vi "test_generic.vi"() -> ()   [LabVIEW 2010, in "GenericObjective.lvclass"]
uses:
  GenericObjective.lvclass
  common/classes/XMLElement/XMLElement/XMLElement.lvclass
  common/classes/GenericComponent/GenericComponent/GenericComponent.lvclass
panel:
  in  "configure button":bool
  in  "stop button":bool
  in  "create OME XML button":bool
  out "OME XML":string
  in  "createButton":bool
  # "Test program for Objective components"
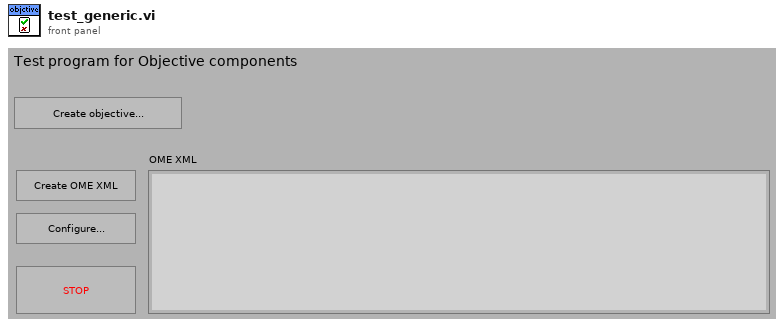
[diagram p1: front panel]
types:
  T1 = typedef "XComponentSpecification.xctl/data.ctl" = cluster{"class path":string, "configuration":string, "label":string, "settings name":string}
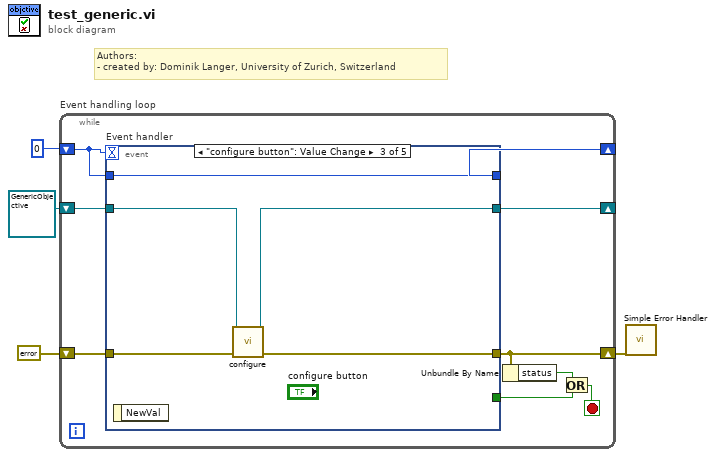
[diagram p0: block diagram]
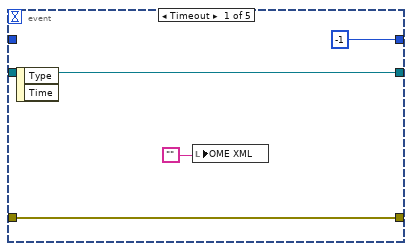
[diagram p2: hidden frame]
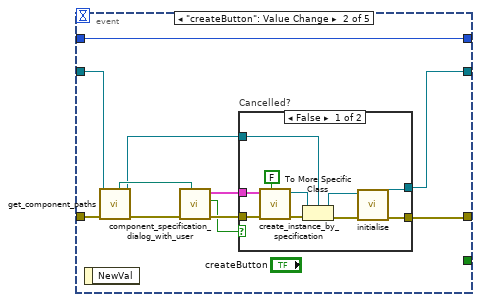
[diagram p3: hidden frame]
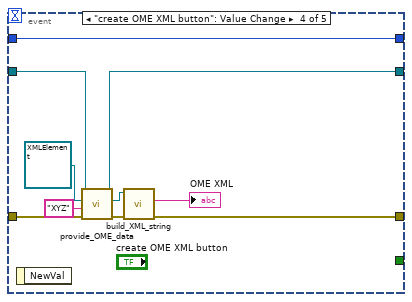
[diagram p5: hidden frame]
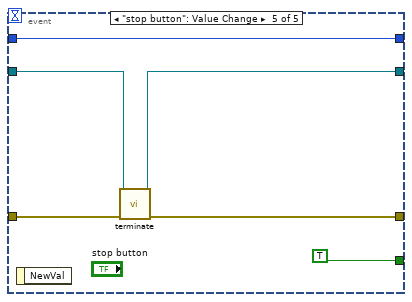
[diagram p6: hidden frame]
diagram:
  # "Authors: \n- created by: Dominik Langer, University of Zurich, Switzerland"
  n1 = while "Event handling loop" {
    shift-right: [w8] -> w1
    shift-left: errorcluster {"status"=FALSE, "code"=0, "source"=""} ("error out") -> [w13]
    shift-right: [w11] -> _
    shift-left: 0 -> [w12]
    shift-right: [w10] -> _
    shift-left: refnum<class "GenericObjective.lvclass"> refnum ("GenericObjective.lvclass") -> [w9]
    stop <- w6 stop-if-true
    n2 = event "Event handler" shown="[2] \"configure button\": Value Change" {
      selector: _ -> [_ _ _ _ _]
      dyn-events: _ -> [_ _ _ _ _]
      timeout: w12 -> [_ _ _ _ _]
      tunnel: w13 -> [w14 w21 w44 w54 w59]
      tunnel: [w14 w27 w43 w47 w58] -> w8
      tunnel: [-1 w28 w45 w55 w61] -> w11
      tunnel: w12 -> [_ w28 w45 w55 w61]
      tunnel: [w15 w26 w41 w52 w56] -> w10
      tunnel: w9 -> [w15 w23 w42 w53 w57]
      tunnel: [_ _ _ _ TRUE] -> w5
      event Timeout {
        n3 = event-data() -> ()  [unwired: 1 in, 2 out]
        n4 = local write "OME XML"("") -> ()
      }
      event "createButton": Value Change {
        n5 = event-data() -> ()  [unwired: 1 in, 1 out]
        n6 = call-dynamic "get_component_paths.vi"("error in (no error)"=w21, "GenericComponent in"=w23) -> ("error out"=w24:errorcluster, "GenericComponent out"=w19:refnum<class "GenericObjective.lvclass">, "component type directory"=w25:path)  [unwired: 4 in, 3 out]
        n7 = call "component_specification_dialog_with_user.vi"("start path"=w25, "error in (no error)"=w24) -> ("error out"=w20:errorcluster, "cancelled?"=w18:bool, "component specification out"=w22:T1)  [unwired: 7 in]
        n8 = case "Cancelled?" shown="False" w18 {
          tunnel: [w38 w40] -> w27
          tunnel: [w37 w39] -> w26
          tunnel: w22 -> [w31 _]
          tunnel: w20 -> [w30 w40]
          tunnel: w19 -> [w29 w39]
          frame False {
            n9 = call "create_instance_by_specification.vi"("call constructor?"=FALSE, "error in (no error)"=w30, "component specification"=w31) -> ("error out"=w33:errorcluster, "GenericPlugin out"=w32:refnum<class "GenericComponent.lvclass">)  [unwired: 6 in, 1 out]
            n10 = To More Specific Class(target class=w29, reference=w32, error in=w33) -> (specific class reference=w35:refnum<class "GenericObjective.lvclass">, error out=w36:errorcluster)
            n11 = call-dynamic "initialise.vi"("error in (no error)"=w36, "GenericPlugin in"=w35) -> ("error out"=w38:errorcluster, "GenericPlugin out"=w37:refnum<class "GenericObjective.lvclass">)  [unwired: 8 in]
          }
          frame True {
          }
        }
      }
      event "configure button": Value Change {
        n12 = event-data() -> ()  [unwired: 1 in, 1 out]
        n13 = call-dynamic "configure.vi"("error in (no error)"=w44, "GenericObjective in"=w42) -> ("error out"=w43:errorcluster, "GenericObjective out"=w41:refnum<class "GenericObjective.lvclass">)  [unwired: 8 in]
      }
      event "create OME XML button": Value Change {
        n14 = event-data() -> ()  [unwired: 1 in, 1 out]
        n15 = call-dynamic "provide_OME_data.vi"("error in (no error)"=w54, "structuredAttribute string in"="XYZ" ("image ID"), "OME element in"=refnum<class "XMLElement.lvclass"> refnum ("XMLElement.lvclass"), "GenericObjective in"=w53) -> ("error out"=w49:errorcluster, "OME element out"=w48:refnum<class "XMLElement.lvclass">, "GenericObjective out"=w52:refnum<class "GenericObjective.lvclass">)  [unwired: 4 in, 1 out]
        n16 = call "build_XML_string.vi"("error in (no error)"=w49, "Element in"=w48) -> ("error out"=w47:errorcluster, "string"=→"OME XML":string)  [unwired: 7 in, 1 out]
      }
      event "stop button": Value Change {
        n17 = event-data() -> ()  [unwired: 1 in, 1 out]
        n18 = call-dynamic "terminate.vi"("error in (no error)"=w59, "GenericPlugin in"=w57) -> ("error out"=w58:errorcluster, "GenericPlugin out"=w56:refnum<class "GenericObjective.lvclass">)  [unwired: 8 in]
      }
    }
    n19 = Unbundle By Name(w8) -> ("status"=w7:bool)
    n20 = Or(x=w7, y=w5) -> (x .or. y?=w6:bool)
  }
  n21 = call <vilib>:"Simple Error Handler.vi"("error in (no error)"=w1) -> ()  [unwired: 4 in, 5 out]
